vi "Terminal-PressureSystem-Getter.vi"(8 "error in (no error)":errorcluster caption="错误输入（无错误）", 11 "read operation timeout (ms)":i32=5000 caption="读操作超时（5000毫秒）") -> (0 "error out":errorcluster caption="错误输出", 2 "时间标识":timestamp, 3 "设备信息":T1)   [LabVIEW 2014]
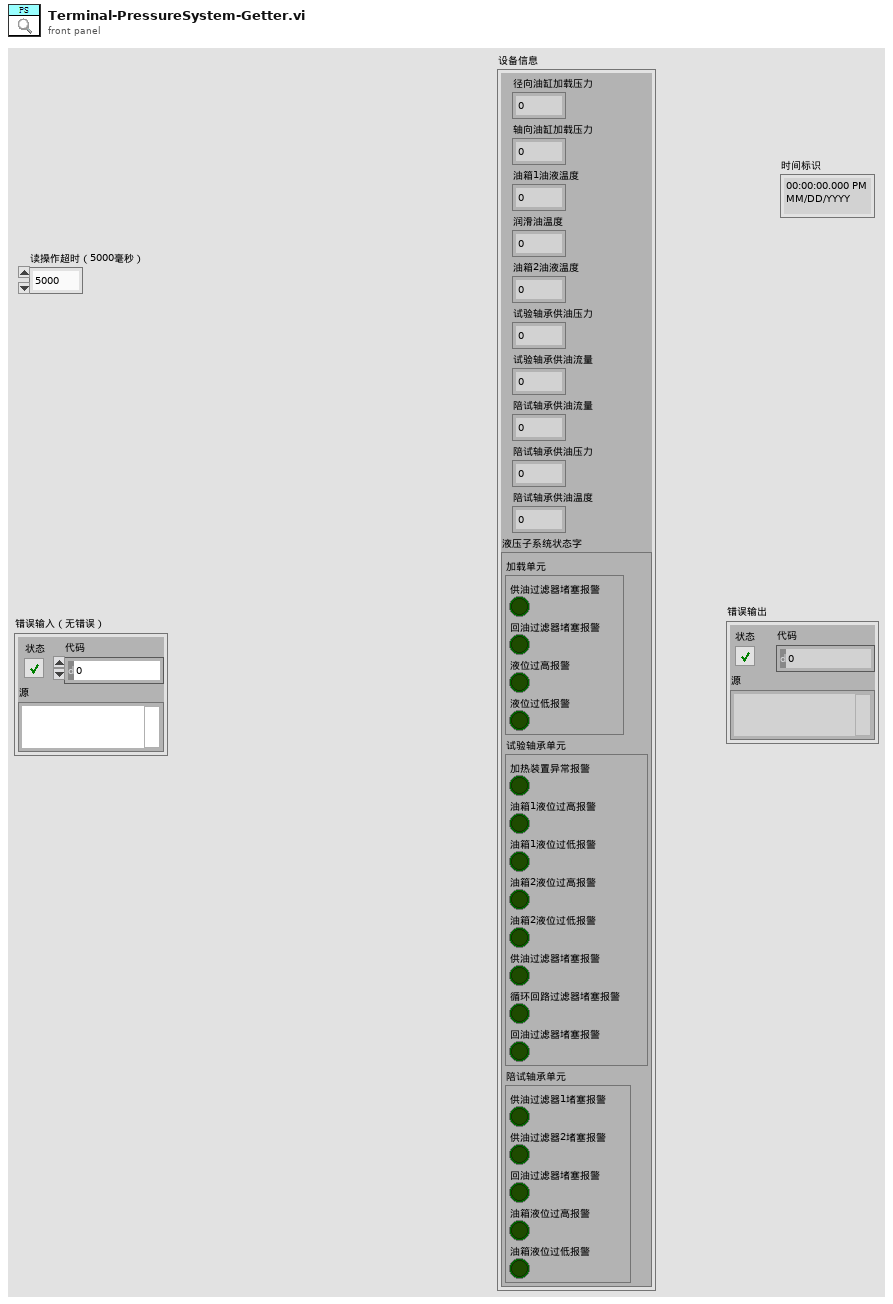
[diagram p1: front panel]
types:
  T1 = cluster{"径向油缸加载压力":u16, "轴向油缸加载压力":u16, "油箱1油液温度":u16, "润滑油温度":u16, "油箱2油液温度":u16, "试验轴承供油压力":u16, "试验轴承供油流量":u16, "陪试轴承供油流量":u16, "陪试轴承供油压力":u16, "陪试轴承供油温度":u16, "液压子系统状态字":cluster{"加载单元":cluster{"供油过滤器堵塞报警":bool, "回油过滤器堵塞报警":bool, "液位过高报警":bool, "液位过低报警":bool}, "试验轴承单元":cluster{"加热装置异常报警":bool, "油箱1液位过高报警":bool, "油箱1液位过低报警":bool, "油箱2液位过高报警":bool, "油箱2液位过低报警":bool, "供油过滤器堵塞报警":bool, "循环回路过滤器堵塞报警":bool, "回油过滤器堵塞报警":bool}, "陪试轴承单元":cluster{"供油过滤器1堵塞报警":bool, "供油过滤器2堵塞报警":bool, "回油过滤器堵塞报警":bool, "油箱液位过高报警":bool, "油箱液位过低报警":bool}}}
  T2 = cluster{"加载单元":cluster{"供油过滤器堵塞报警":bool, "回油过滤器堵塞报警":bool, "液位过高报警":bool, "液位过低报警":bool}, "试验轴承单元":cluster{"加热装置异常报警":bool, "油箱1液位过高报警":bool, "油箱1液位过低报警":bool, "油箱2液位过高报警":bool, "油箱2液位过低报警":bool, "供油过滤器堵塞报警":bool, "循环回路过滤器堵塞报警":bool, "回油过滤器堵塞报警":bool}, "陪试轴承单元":cluster{"供油过滤器1堵塞报警":bool, "供油过滤器2堵塞报警":bool, "回油过滤器堵塞报警":bool, "油箱液位过高报警":bool, "油箱液位过低报警":bool}}
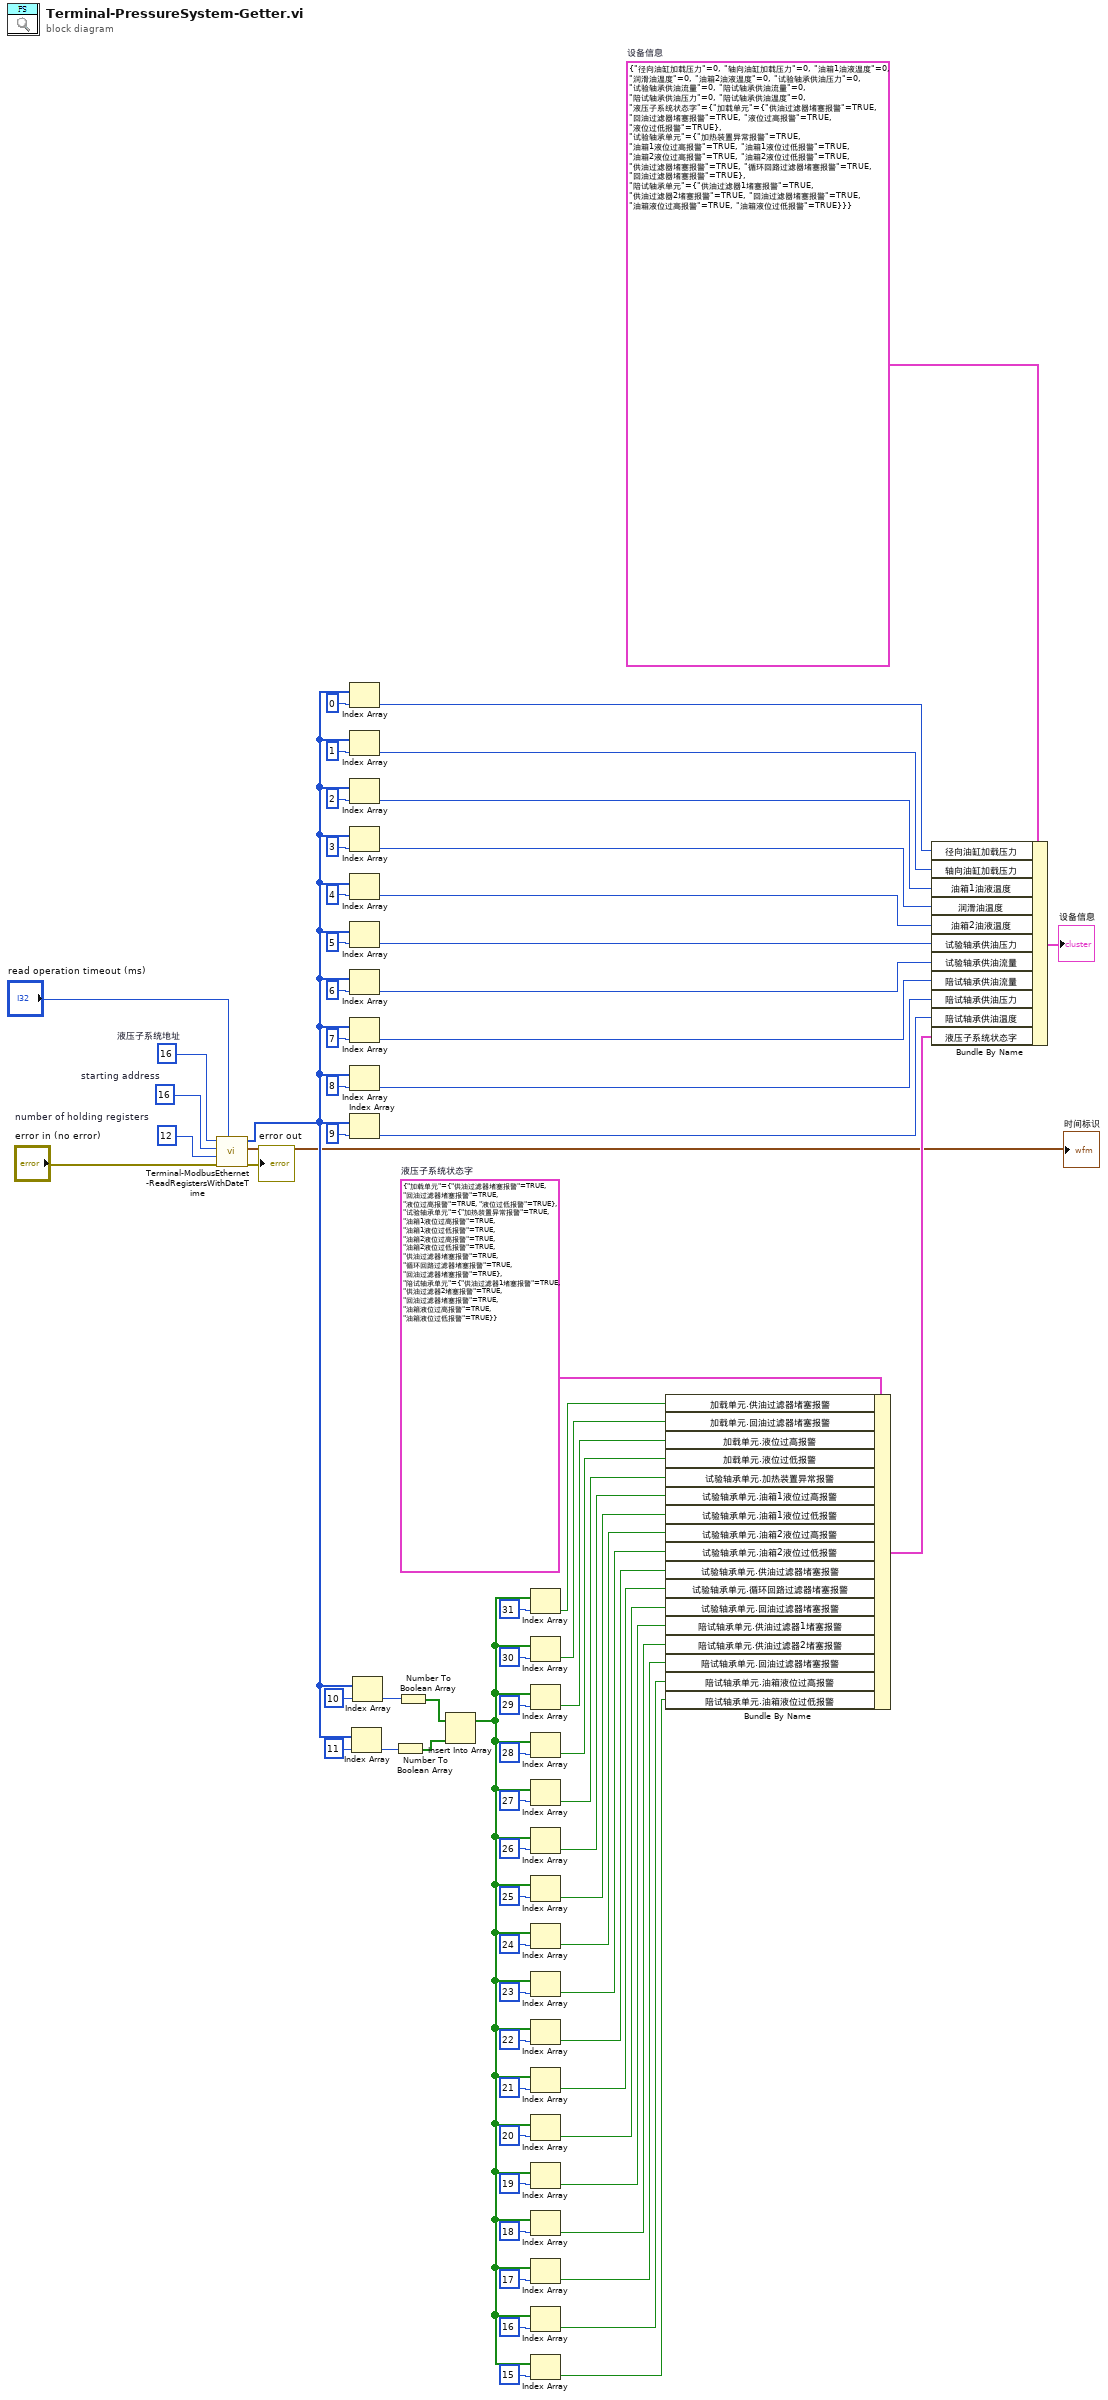
[diagram p0: block diagram]
diagram:
  w21 = T2 {"加载单元"={"供油过滤器堵塞报警"=TRUE, "回油过滤器堵塞报警"=TRUE, "液位过高报警"=TRUE, "液位过低报警"=TRUE}, "试验轴承单元"={"加热装置异常报警"=TRUE, "油箱1液位过高报警"=TRUE, "油箱1液位过低报警"=TRUE, "油箱2液位过高报警"=TRUE, "油箱2液位过低报警"=TRUE, "供油过滤器堵塞报警"=TRUE, "循环回路过滤器堵塞报警"=TRUE, "回油过滤器堵塞报警"=TRUE}, "陪试轴承单元"={"供油过滤器1堵塞报警"=TRUE, "供油过滤器2堵塞报警"=TRUE, "回油过滤器堵塞报警"=TRUE, "油箱液位过高报警"=TRUE, "油箱液位过低报警"=TRUE}}  # 液压子系统状态字
  w67 = T1 {"径向油缸加载压力"=0, "轴向油缸加载压力"=0, "油箱1油液温度"=0, "润滑油温度"=0, "油箱2油液温度"=0, "试验轴承供油压力"=0, "试验轴承供油流量"=0, "陪试轴承供油流量"=0, "陪试轴承供油压力"=0, "陪试轴承供油温度"=0, "液压子系统状态字"={"加载单元"={"供油过滤器堵塞报警"=TRUE, "回油过滤器堵塞报警"=TRUE, "液位过高报警"=TRUE, "液位过低报警"=TRUE}, "试验轴承单元"={"加热装置异常报警"=TRUE, "油箱1液位过高报警"=TRUE, "油箱1液位过低报警"=TRUE, "油箱2液位过高报警"=TRUE, "油箱2液位过低报警"=TRUE, "供油过滤器堵塞报警"=TRUE, "循环回路过滤器堵塞报警"=TRUE, "回油过滤器堵塞报警"=TRUE}, "陪试轴承单元"={"供油过滤器1堵塞报警"=TRUE, "供油过滤器2堵塞报警"=TRUE, "回油过滤器堵塞报警"=TRUE, "油箱液位过高报警"=TRUE, "油箱液位过低报警"=TRUE}}}  # 设备信息
  w71 = u16 12  # number of holding registers
  w72 = u16 16  # starting address
  w73 = u8 16  # 液压子系统地址
  n1 = call "Terminal-ModbusEthernet-ReadRegistersWithDateTime.vi"("read operation timeout (ms)"="read operation timeout (ms)", "error in"="error in (no error)", "number of holding registers"=w71, "starting address"=w72, "unit ID"=w73) -> ("error out"=→"error out":errorcluster, "时间标识"=→"时间标识":timestamp, "register values"=w8:u16[])  [unwired: 4 in]
  n2 = Index Array(array=w8, index=0 ("索引")) -> (element=w65:u16)
  n3 = Index Array(array=w8, index=1 ("索引")) -> (element=w61:u16)
  n4 = Index Array(array=w8, index=2 ("索引")) -> (element=w60:u16)
  n5 = Index Array(array=w8, index=3 ("索引")) -> (element=w59:u16)
  n6 = Index Array(array=w8, index=4 ("索引")) -> (element=w44:u16)
  n7 = Index Array(array=w8, index=5 ("索引")) -> (element=w43:u16)
  n8 = Index Array(array=w8, index=6 ("索引")) -> (element=w42:u16)
  n9 = Index Array(array=w8, index=7 ("索引")) -> (element=w41:u16)
  n10 = Index Array(array=w8, index=8 ("索引")) -> (element=w40:u16)
  n11 = Index Array(array=w8, index=9 ("索引")) -> (element=w39:u16)
  n12 = Index Array(array=w8, index=11 ("索引")) -> (element=w5:u16)
  n13 = Index Array(array=w8, index=10 ("索引")) -> (element=w6:u16)
  n14 = Number To Boolean Array(number=w5) -> (Boolean array=w3:bool[])
  n15 = Number To Boolean Array(number=w6) -> (Boolean array=w4:bool[])
  n16 = Insert Into Array(array=w4, new element=w3) -> (w2:bool[])  [unwired: 1 in]
  n17 = Index Array(array=w2, index=31 ("索引")) -> (element=w54:bool)
  n18 = Index Array(array=w2, index=30 ("索引")) -> (element=w53:bool)
  n19 = Index Array(array=w2, index=29 ("索引")) -> (element=w52:bool)
  n20 = Index Array(array=w2, index=28 ("索引")) -> (element=w51:bool)
  n21 = Index Array(array=w2, index=27 ("索引")) -> (element=w31:bool)
  n22 = Index Array(array=w2, index=26 ("索引")) -> (element=w30:bool)
  n23 = Index Array(array=w2, index=25 ("索引")) -> (element=w29:bool)
  n24 = Index Array(array=w2, index=24 ("索引")) -> (element=w28:bool)
  n25 = Index Array(array=w2, index=23 ("索引")) -> (element=w27:bool)
  n26 = Index Array(array=w2, index=22 ("索引")) -> (element=w26:bool)
  n27 = Index Array(array=w2, index=21 ("索引")) -> (element=w23:bool)
  n28 = Index Array(array=w2, index=20 ("索引")) -> (element=w22:bool)
  n29 = Index Array(array=w2, index=19 ("索引")) -> (element=w14:bool)
  n30 = Index Array(array=w2, index=18 ("索引")) -> (element=w13:bool)
  n31 = Index Array(array=w2, index=17 ("索引")) -> (element=w12:bool)
  n32 = Index Array(array=w2, index=16 ("索引")) -> (element=w11:bool)
  n33 = Index Array(array=w2, index=15 ("索引")) -> (element=w10:bool)
  n34 = Bundle By Name(cluster=w21, "加载单元.供油过滤器堵塞报警"=w54, "加载单元.回油过滤器堵塞报警"=w53, "加载单元.液位过高报警"=w52, "加载单元.液位过低报警"=w51, "试验轴承单元.加热装置异常报警"=w31, "试验轴承单元.油箱1液位过高报警"=w30, "试验轴承单元.油箱1液位过低报警"=w29, "试验轴承单元.油箱2液位过高报警"=w28, "试验轴承单元.油箱2液位过低报警"=w27, "试验轴承单元.供油过滤器堵塞报警"=w26, "试验轴承单元.循环回路过滤器堵塞报警"=w23, "试验轴承单元.回油过滤器堵塞报警"=w22, "陪试轴承单元.供油过滤器1堵塞报警"=w14, "陪试轴承单元.供油过滤器2堵塞报警"=w13, "陪试轴承单元.回油过滤器堵塞报警"=w12, "陪试轴承单元.油箱液位过高报警"=w11, "陪试轴承单元.油箱液位过低报警"=w10) -> (w38:T2)
  n35 = Bundle By Name(cluster=w67, "径向油缸加载压力"=w65, "轴向油缸加载压力"=w61, "油箱1油液温度"=w60, "润滑油温度"=w59, "油箱2油液温度"=w44, "试验轴承供油压力"=w43, "试验轴承供油流量"=w42, "陪试轴承供油流量"=w41, "陪试轴承供油压力"=w40, "陪试轴承供油温度"=w39, "液压子系统状态字"=w38) -> (→"设备信息":T1)
